vi "Debug_Convert_Data_to_String.vi"(8 "error in (no error)":errorcluster, 11 "AB_Deploy_EXE in":refnum<class "AB_Deploy_EXE.lvclass">) -> (0 "error out":errorcluster, 2 "classData":string, 3 "AB_Deploy_EXE out":refnum<class "AB_Deploy_EXE.lvclass">)   [LabVIEW 2020, in "AB_Deploy_EXE.lvclass"]
uses:
  <vilib>/AppBuilder/AB_Classes/DeployableEXE/AB_Deploy_EXE.lvclass
  <vilib>/AppBuilder/AB_Classes/DeployableEXE/AB_Deploy_EXE.lvclass/AB_Deploy_EXE.ctl
  <vilib>/AppBuilder/AB_Classes/EXE/AB_EXE.lvclass
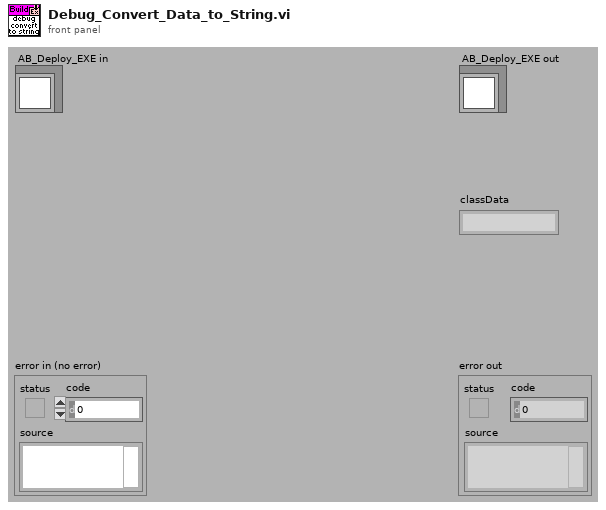
[diagram p1: front panel]
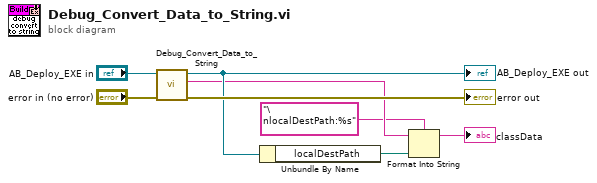
[diagram p0: block diagram]
diagram:
  n1 = call-parent "Debug_Convert_Data_to_String.vi"("error in (no error)"="error in (no error)", "AB_EXE in"="AB_Deploy_EXE in") -> ("error out"=→"error out":errorcluster, "classData"=w4:string, "AB_EXE out"=w5:refnum<class "AB_Deploy_EXE.lvclass">)  [unwired: 7 in]
  "AB_Deploy_EXE out" <- w5
  n2 = Unbundle By Name(w5) -> ("localDestPath"=w2:path)
  n3 = Format Into String(format string="\nlocalDestPath:%s", initial string=w4, w2) -> (resulting string=→"classData":string)  [unwired: 1 in, 1 out]
